vi "__parseConfiguration.vi"(8 "error in":errorcluster, 11 "configFilePath":path) -> (0 "error out":errorcluster, 3 "room_map":map{string, T1}(c390))   [LabVIEW 2020, in "Room-API.lvclass"]
uses:
  Room-API.lvclass
  Single Room.ctl
  b2d56093-1e09-4035-af7c-025cfe40be0f.vi
  <vilib>/JDP Science/JSONtext/String Subset.vi
  <vilib>/JDP Science/JSONtext/Parsing/Parse Full Path or Item Name.vi
  <vilib>/JDP Science/JSONtext/Offset/Find Item Locations by Path.vi
  <vilib>/JDP Science/JSONtext/JSON text to Variant.vi
  <vilib>/JDP Science/JSONtext/JSONtext.lvlib
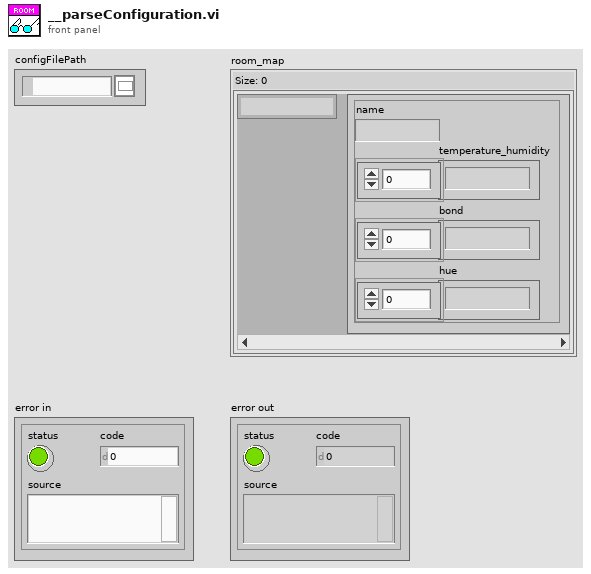
[diagram p1: front panel]
types:
  T1 = typedef "Room-API.lvclass/Single Room.ctl" = cluster{"name":string, "temperature_humidity":string[], "bond":string[], "hue":string[]}
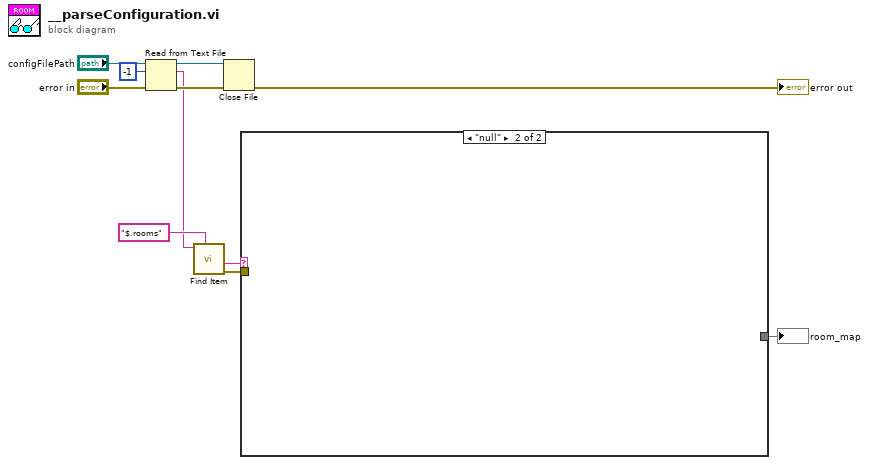
[diagram p0: block diagram]
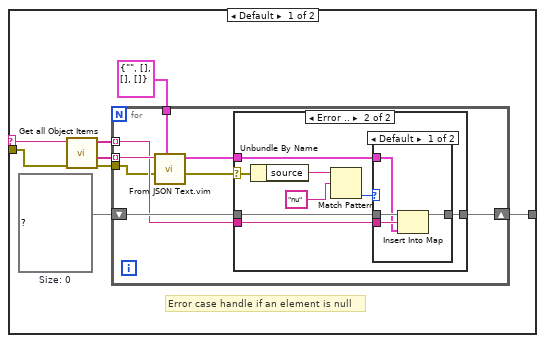
[diagram p2: hidden frame]
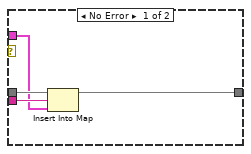
[diagram p3: hidden frame]
diagram:
  n1 = Read from Text File(file (use dialog)="configFilePath", count=-1, error in="error in") -> (refnum out=w6:refnum<file>, text=w3:string, error out=w5:errorcluster)  [unwired: 1 in, 1 out]
  n2 = call <vilib>:"Find Item.vi"("$Path or Item Name"="$.rooms", "JSON"=w3) -> ("error out"=w9:errorcluster, "<JSON>"=w10:string)  [unwired: 6 in, 2 out]
  n3 = Close File(refnum=w6, error in=w5) -> (error out=→"error out":errorcluster)  [unwired: 1 out]
  n4 = case shown="\"null\"" w10 {
    selector: w10 -> [w19 _]
    tunnel: w9 -> [w14 _]
    tunnel: [w12 _] -> w1
    frame Default {
      w15 = map{string, T1} {}  # Size: 0
      # "Error case handle if an element is null"
      n5 = call <vilib>:"Get all Object Items.vi"("error in (no error)"=w14, "JSON"=w19) -> ("error out"=w13:errorcluster, "<JSON>"=w17:string[], "Item Names"=w18:string[])  [unwired: 6 in, 1 out]
      n6 = for {
        tunnel: w18 -> [w24] mode=indexing
        tunnel: w17 -> [w27] mode=indexing
        tunnel: T1 {"name"="", "temperature_humidity"=[], "bond"=[], "hue"=[]} ("singleRoom") -> [w26]
        shift-right: [w23] -> w12
        shift-left: w15 -> [w25]
        tunnel: w13 -> [w20]
        n7 = call "From JSON Text.vim"("Data Type and Default Value"=w26, "error in (no error)"=w20, "JSON"=w27) -> ("error out"=w21:errorcluster, "Data out"=w22:T1)  [unwired: 7 in]
        n8 = case shown="Error .." w21 {
          selector: w21 -> [_ w39]
          tunnel: w25 -> [w31 w35]
          tunnel: w24 -> [w30 w34]
          tunnel: [w29 w33] -> w23
          tunnel: w22 -> [w28 w32]
          frame No Error {
            n9 = Insert Into Map(map in=w31, key=w30, value=w28) -> (map out=w29:map{string, T1})  [unwired: 2 out]
          }
          frame Error {
            n10 = Unbundle By Name(w39) -> ("source"=w38:string)
            n11 = Match Pattern(string=w38, regular expression="nu") -> (offset past match=w36:i32)  [unwired: 1 in, 3 out]
            n12 = case shown="Default" w36 {
              tunnel: w35 -> [w43 w44]
              tunnel: w34 -> [w41 _]
              tunnel: [w42 w44] -> w33
              tunnel: w32 -> [w40 _]
              frame Default {
                n13 = Insert Into Map(map in=w43, key=w41, value=w40) -> (map out=w42:map{string, T1})  [unwired: 2 out]
              }
              frame -1 {
              }
            }
          }
        }
      }
    }
    frame "null" {
    }
  }
  "room_map" <- w1
